vi "AverageOneCoord (SubVI).vi"(0 "Array":dbl[](array[numeric])) -> (4 "Top averages":dbl[][](array[numeric]), 6 "Bottom averages":dbl[][](array[numeric]), 8 "Top SD":dbl[][](array[numeric]), 10 "Bottom SD":dbl[][](array[numeric]))   [LabVIEW 2016]
uses:
  <vilib>/Analysis/NI_AALBase.lvlib
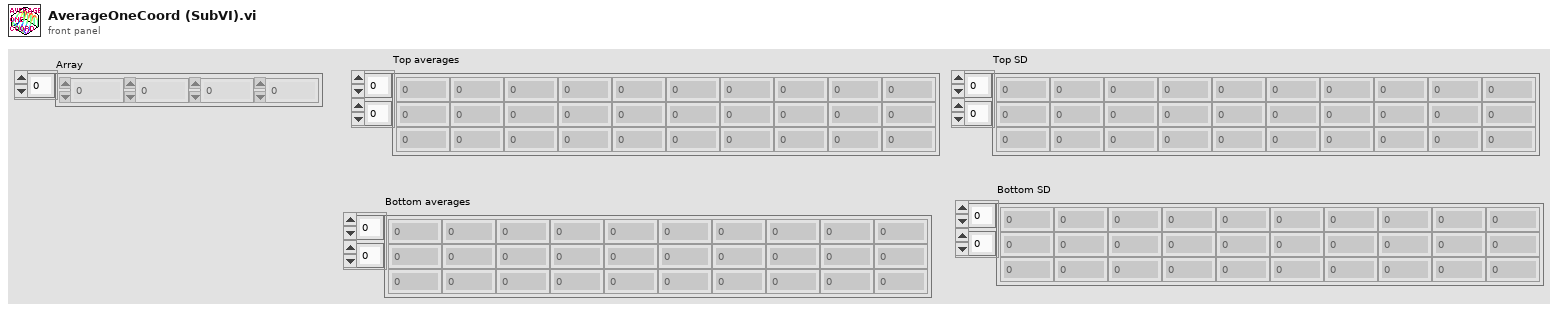
[diagram p1: front panel]
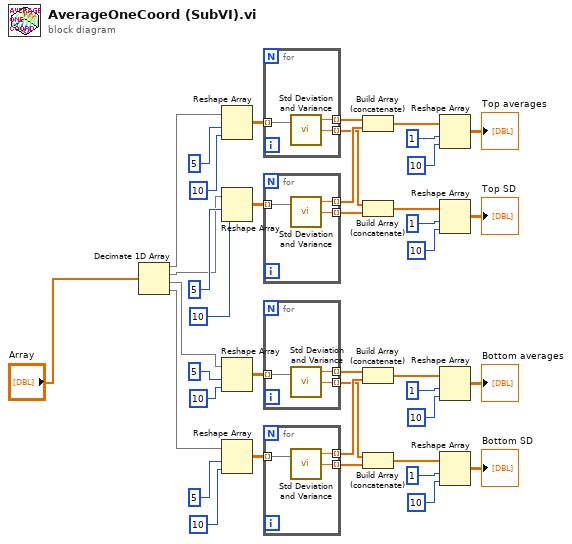
[diagram p0: block diagram]
diagram:
  n1 = Decimate 1D Array("Array") -> (w39:dbl[], w33:dbl[], w29:dbl[], w25:dbl[])
  n2 = Reshape Array(w39, 5 ("dimension size"), 10 ("dimension size")) -> (w37:dbl[][])
  n3 = Reshape Array(w33, 5 ("dimension size"), 10 ("dimension size")) -> (w34:dbl[][])
  n4 = Reshape Array(w29, 5 ("dimension size"), 10 ("dimension size")) -> (w30:dbl[][])
  n5 = Reshape Array(w25, 5 ("dimension size"), 10 ("dimension size")) -> (w26:dbl[][])
  n6 = for {
    tunnel: w37 -> [w44] mode=indexing
    tunnel: [w43] -> w24 mode=indexing
    tunnel: [w42] -> w6 mode=indexing
    n7 = call <vilib>:"Std Deviation and Variance.vi"("X"=w44) -> ("mean"=w43:dbl, "standard deviation"=w42:dbl)  [unwired: 1 in, 1 out]
  }
  n8 = for {
    tunnel: w34 -> [w47] mode=indexing
    tunnel: [w46] -> w23 mode=indexing
    tunnel: [w45] -> w5 mode=indexing
    n9 = call <vilib>:"Std Deviation and Variance.vi"("X"=w47) -> ("mean"=w46:dbl, "standard deviation"=w45:dbl)  [unwired: 1 in, 1 out]
  }
  n10 = for {
    tunnel: w30 -> [w50] mode=indexing
    tunnel: [w49] -> w4 mode=indexing
    tunnel: [w48] -> w2 mode=indexing
    n11 = call <vilib>:"Std Deviation and Variance.vi"("X"=w50) -> ("mean"=w49:dbl, "standard deviation"=w48:dbl)  [unwired: 1 in, 1 out]
  }
  n12 = for {
    tunnel: w26 -> [w53] mode=indexing
    tunnel: [w52] -> w3 mode=indexing
    tunnel: [w51] -> w1 mode=indexing
    n13 = call <vilib>:"Std Deviation and Variance.vi"("X"=w53) -> ("mean"=w52:dbl, "standard deviation"=w51:dbl)  [unwired: 1 in, 1 out]
  }
  n14 = Build Array (concatenate)(w24, w23) -> (w22:dbl[])
  n15 = Build Array (concatenate)(w6, w5) -> (w18:dbl[])
  n16 = Build Array (concatenate)(w4, w3) -> (w14:dbl[])
  n17 = Build Array (concatenate)(w2, w1) -> (w10:dbl[])
  n18 = Reshape Array(w22, 1 ("dimension size"), 10 ("dimension size")) -> (→"Top averages":dbl[][])
  n19 = Reshape Array(w18, 1 ("dimension size"), 10 ("dimension size")) -> (→"Top SD":dbl[][])
  n20 = Reshape Array(w14, 1 ("dimension size"), 10 ("dimension size")) -> (→"Bottom averages":dbl[][])
  n21 = Reshape Array(w10, 1 ("dimension size"), 10 ("dimension size")) -> (→"Bottom SD":dbl[][])
